vi "Untitled 1.vi"() -> ()   [LabVIEW 2018]
uses:
  <instrlib>/niDCPower/nidcpower.llb/niDCPower Source Mode.ctl
  <instrlib>/niDCPower/nidcpower.llb/niDCPower Output Function.ctl
panel:
  in  "voltage level range 2":dbl=-2.0 caption="voltage level range" format="%.6p"
  in  "voltage level range 0":dbl=2.0 caption="voltage level range" format="%.6p"
  out "I2":dbl=-1.8616481828800653e-06
  out "V2":dbl=0.000859850971924123
  out "I0":dbl=6.67426339573744e-05
  out "V0":dbl=-7.674732610793108e-05
  out "Power off":bool=TRUE
  in  "POWER":bool
  in  "voltlim_I_LED, V":dbl=2.0 caption="current limit" min=0.01 format="%_6p"
  in  "I_LED, A":dbl=0.005 caption="voltage level" format="%_6p"
  in  "V_MB, V":dbl=4.0 caption="voltage level" format="%_6p"
  in  "curlim_V_MB, A":dbl=0.01 caption="current limit" format="%_6p"
  in  "curlim_V_RES, A":dbl=0.1 caption="current limit" min=0.01 format="%_6p"
  in  "V_RES, V":dbl=-2.0 caption="voltage level" format="%_6p"
  in  "current level range 1":dbl=0.007 caption="current level range" format="%#.6p"
  out "V1":dbl=2.9889440267337464e-05
  out "I1":dbl=1.0159805781779444e-06
  in  "Стоп":bool
  in  "Resource Name":refnum<k15>="PXI1Slot2" caption="Источник питания"
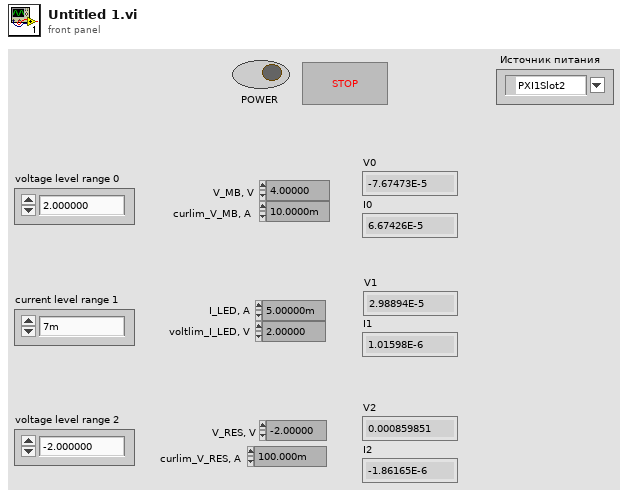
[diagram p1: front panel]
types:
  T1 = typedef "niDCPower Output Function.ctl" = i32
  T2 = typedef "niDCPower Source Mode.ctl" = i32
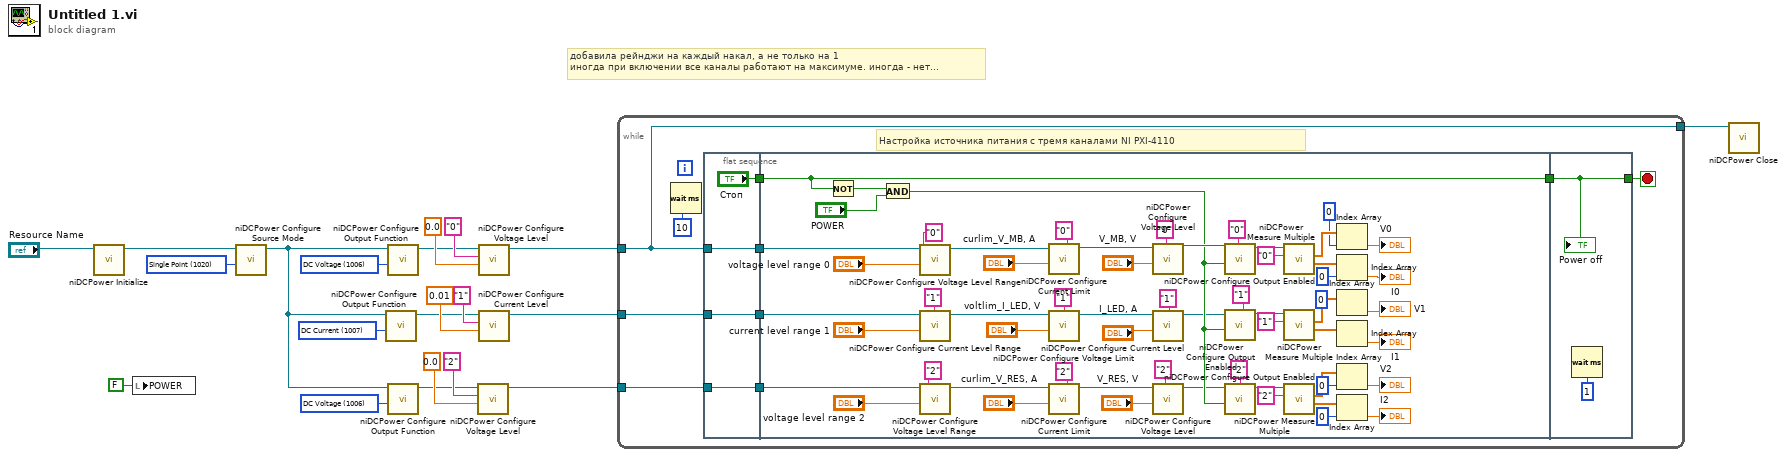
[diagram p0: block diagram]
diagram:
  w4 = T1 1006 items=["DC Voltage"=1006, "DC Current"=1007, "Pulse Voltage"=1049, "Pulse Current"=1050] ("output function")
  w11 = T1 1007 items=["DC Voltage"=1006, "DC Current"=1007, "Pulse Voltage"=1049, "Pulse Current"=1050] ("output function")
  w12 = T1 1006 items=["DC Voltage"=1006, "DC Current"=1007, "Pulse Voltage"=1049, "Pulse Current"=1050] ("output function")
  w15 = T2 1020 items=["Single Point"=1020, "Sequence"=1021] ("source mode")
  # "добавила рейнджи на каждый накал, а не только на 1\nиногда при включении все каналы работают на максимуме. иногда - нет..."
  n1 = call <instrlib>:"niDCPower Initialize.vi"("resource name"="Resource Name") -> ("instrument handle out"=w16:refnum<k15>)  [unwired: 3 in, 7 out]
  n2 = local write "POWER"(FALSE ("POWER")) -> ()
  n3 = call <instrlib>:"niDCPower Configure Source Mode.vi"("source mode"=w15, "instrument handle"=w16) -> ("instrument handle out"=w3:refnum<k15>)  [unwired: 1 in, 8 out]
  n4 = call <instrlib>:"niDCPower Configure Output Function.vi"("output function"=w11, "instrument handle"=w3) -> ("instrument handle out"=w13:refnum<k15>)  [unwired: 8 in, 1 out]
  n5 = call <instrlib>:"niDCPower Configure Output Function.vi"("output function"=w12, "instrument handle"=w3) -> ("instrument handle out"=w14:refnum<k15>)  [unwired: 8 in, 1 out]
  n6 = call <instrlib>:"niDCPower Configure Output Function.vi"("output function"=w4, "instrument handle"=w3) -> ("instrument handle out"=w5:refnum<k15>)  [unwired: 8 in, 1 out]
  n7 = call <instrlib>:"niDCPower Configure Voltage Level.vi"("voltage level"=0.0, "channel name"="2", "instrument handle"=w5) -> ("instrument handle out"=w2:refnum<k15>)  [unwired: 7 in, 1 out]
  n8 = call <instrlib>:"niDCPower Configure Voltage Level.vi"("voltage level"=0.0, "channel name"="0", "instrument handle"=w14) -> ("instrument handle out"=w8:refnum<k15>)  [unwired: 7 in, 1 out]
  n9 = call <instrlib>:"niDCPower Configure Current Level.vi"("current level"=0.01, "channel name"="1", "instrument handle"=w13) -> ("instrument handle out"=w9:refnum<k15>)  [unwired: 7 in, 1 out]
  n10 = while {
    tunnel: w8 -> [w28]
    tunnel: [w28] -> w10
    tunnel: w9 -> [w25]
    tunnel: w2 -> [w22]
    stop <- w24 stop-if-true
    # "Настройка источника питания с тремя каналами NI PXI-4110"
    n11 = Wait (ms)(milliseconds to wait=u32 10) -> ()  [unwired: 1 out]
    n12 = flat-sequence {
      tunnel: w28 -> [w35]
      tunnel: [w35] -> w30
      tunnel: ["Стоп"] -> w29
      tunnel: [w33] -> w26
      tunnel: w25 -> [w33]
      tunnel: [w32] -> w23
      tunnel: w22 -> [w32]
      tunnel: w30 -> [w43]
      tunnel: w29 -> [w95]
      tunnel: [w95] -> w27
      tunnel: w26 -> [w60]
      tunnel: w23 -> [w41]
      tunnel: [w97] -> w24
      tunnel: w27 -> [w97]
      frame #0 {
      }
      frame #1 {
        n13 = Not(x=w95) -> (.not. x?=w94:bool)
        n14 = And(x=w94, y="POWER") -> (x .and. y?=w91:bool)
        n15 = call <instrlib>:"niDCPower Configure Voltage Level Range.vi"("voltage level range"="voltage level range 0", "channel name"="0", "instrument handle"=w43) -> ("instrument handle out"=w42:refnum<k15>)  [unwired: 7 in, 1 out]
        n16 = call <instrlib>:"niDCPower Configure Current Level Range.vi"("current level range"="current level range 1", "channel name"="1", "instrument handle"=w60) -> ("instrument handle out"=w59:refnum<k15>)  [unwired: 7 in, 1 out]
        n17 = call <instrlib>:"niDCPower Configure Voltage Level Range.vi"("voltage level range"="voltage level range 2", "channel name"="2", "instrument handle"=w41) -> ("instrument handle out"=w40:refnum<k15>)  [unwired: 7 in, 1 out]
        n18 = call <instrlib>:"niDCPower Configure Current Limit.vi"("current limit"="curlim_V_MB, A", "channel name"="0", "instrument handle"=w42) -> ("instrument handle out"=w82:refnum<k15>)  [unwired: 7 in, 1 out]
        n19 = call <instrlib>:"niDCPower Configure Voltage Limit.vi"("voltage limit"="voltlim_I_LED, V", "channel name"="1", "instrument handle"=w59) -> ("instrument handle out"=w86:refnum<k15>)  [unwired: 7 in, 1 out]
        n20 = call <instrlib>:"niDCPower Configure Current Limit.vi"("current limit"="curlim_V_RES, A", "channel name"="2", "instrument handle"=w40) -> ("instrument handle out"=w76:refnum<k15>)  [unwired: 7 in, 1 out]
        n21 = call <instrlib>:"niDCPower Configure Voltage Level.vi"("voltage level"="V_MB, V", "channel name"="0", "instrument handle"=w82) -> ("instrument handle out"=w92:refnum<k15>)  [unwired: 7 in, 1 out]
        n22 = call <instrlib>:"niDCPower Configure Current Level.vi"("current level"="I_LED, A", "channel name"="1", "instrument handle"=w86) -> ("instrument handle out"=w87:refnum<k15>)  [unwired: 7 in, 1 out]
        n23 = call <instrlib>:"niDCPower Configure Voltage Level.vi"("voltage level"="V_RES, V", "channel name"="2", "instrument handle"=w76) -> ("instrument handle out"=w77:refnum<k15>)  [unwired: 7 in, 1 out]
        n24 = call <instrlib>:"niDCPower Configure Output Enabled.vi"("output enabled"=w91, "channel name"="0", "instrument handle"=w92) -> ("instrument handle out"=w70:refnum<k15>)  [unwired: 7 in, 1 out]
        n25 = call <instrlib>:"niDCPower Configure Output Enabled.vi"("output enabled"=w91, "channel name"="1", "instrument handle"=w87) -> ("instrument handle out"=w63:refnum<k15>)  [unwired: 7 in, 1 out]
        n26 = call <instrlib>:"niDCPower Configure Output Enabled.vi"("output enabled"=w91, "channel name"="2", "instrument handle"=w77) -> ("instrument handle out"=w62:refnum<k15>)  [unwired: 7 in, 1 out]
        n27 = call <instrlib>:"niDCPower Measure Multiple.vi"("channel name"="0", "instrument handle"=w70) -> ("current measurements"=w68:dbl[], "voltage measurements"=w69:dbl[])  [unwired: 6 in, 2 out]
        n28 = call <instrlib>:"niDCPower Measure Multiple.vi"("channel name"="1", "instrument handle"=w63) -> ("current measurements"=w66:dbl[], "voltage measurements"=w67:dbl[])  [unwired: 6 in, 2 out]
        n29 = call <instrlib>:"niDCPower Measure Multiple.vi"("channel name"="2", "instrument handle"=w62) -> ("current measurements"=w64:dbl[], "voltage measurements"=w65:dbl[])  [unwired: 6 in, 2 out]
        n30 = Index Array(array=w69, index=0) -> (element=→"V0":dbl)
        n31 = Index Array(array=w68, index=0) -> (element=→"I0":dbl)
        n32 = Index Array(array=w67, index=0) -> (element=→"V1":dbl)
        n33 = Index Array(array=w66) -> (element=→"I1":dbl)  [unwired: 1 in]
        n34 = Index Array(array=w65, index=0) -> (element=→"V2":dbl)
        n35 = Index Array(array=w64, index=0) -> (element=→"I2":dbl)
      }
      frame #2 {
        n36 = Wait (ms)(milliseconds to wait=u32 1) -> ()  [unwired: 1 out]
        "Power off" <- w97
      }
    }
  }
  n37 = call <instrlib>:"niDCPower Close.vi"("instrument handle"=w10) -> ()  [unwired: 10 in, 1 out]
